vi "Manual Assembly DB.vi"() -> ()   [LabVIEW 2021]
uses:
  Classes/Routine/Routine Enum.ctl
  Classes/Assembly/Database Entry/Database Entry.lvclass
  Classes/Assembly/Assembly Run.lvclass
  Classes/Workspace/Fixture Enum.ctl
  Classes/Controller/Controller.lvclass
  Classes/Workspace/Fixture.lvclass
  Classes/Routine/Routine.lvclass
panel:
  in  "Type":bool
  out "String":string
  in  "Clear All":bool
  in  "Assemble":bool
  in  "Dispense offset":bool
  in  "Pick and Place":bool
  in  "Dispense glue":bool
  in  "Go":bool
  in  "Routine":T1=enum."Dispense on Plate"
  in  "Update":bool
  in  "Stage":i32(listbox)=-1
  in  "Stop":bool
  in  "Remove":bool
  in  "Add":bool
  # "Protomodule"
  # "Module"
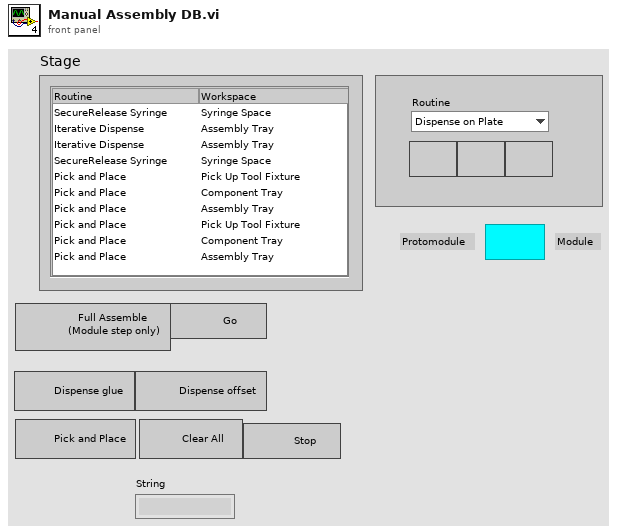
[diagram p1: front panel]
types:
  T1 = typedef "Routine.lvclass/Routine Enum.ctl" = enum16{"Primary Pick Up", "Pick Up All", "Put Down Secondary", "Put Down All", "Release Syringe", "Secondary Pick Up", "Secure Syringe", "Dispense on Plate", "Dispense on Kapton", "Dispense on Sensor"}
  T2 = typedef "Fixture.lvclass/Fixture Enum.ctl" = enum16{"Assembly Tray", "Syringe Space", "Component", "Pick Up Tool", "Current Position"}
  T3 = typedef "Controller.lvclass/Controllers.ctl" = cluster{"I-O.lvclass":refnum<class "I-O.lvclass">, "Gantry":refnum<k24>, "Dispenser":refnum<visa-resource-name>}
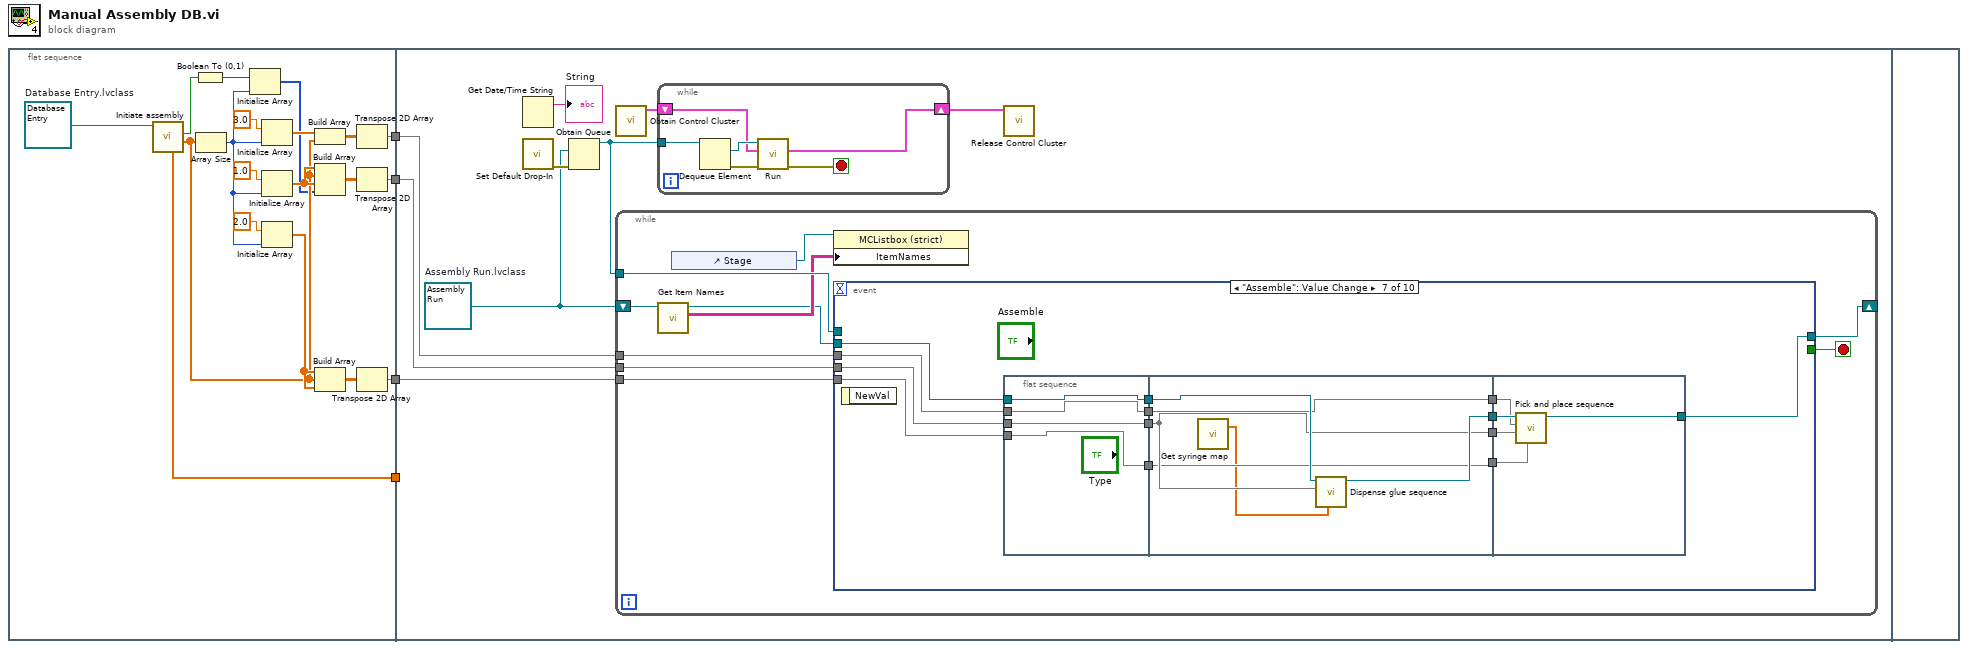
[diagram p0: block diagram]
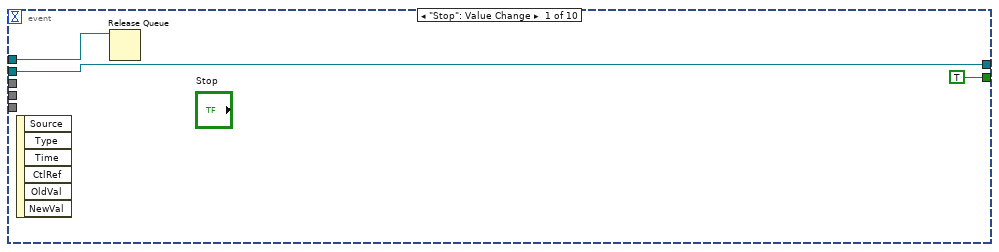
[diagram p2: hidden frame]
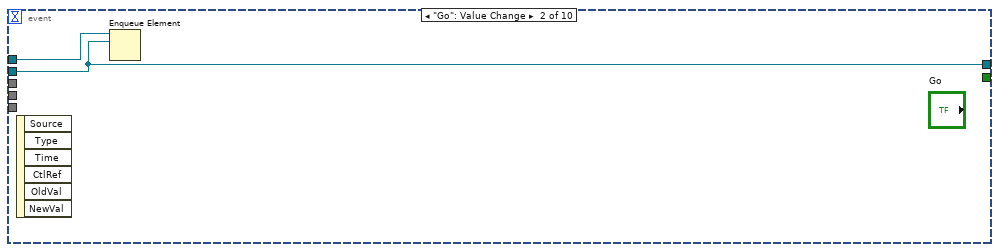
[diagram p3: hidden frame]
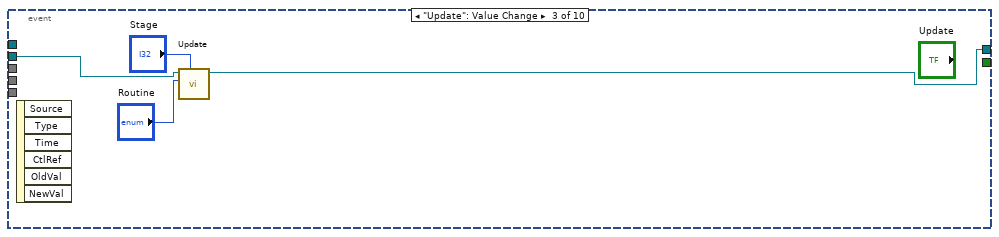
[diagram p4: hidden frame]
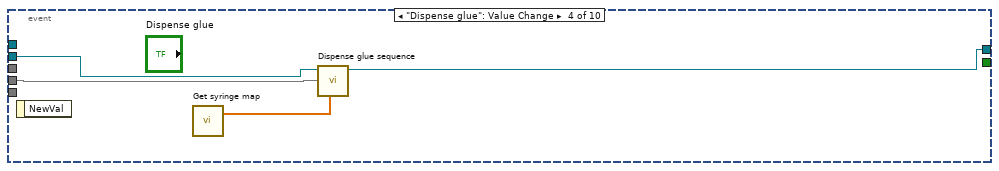
[diagram p5: hidden frame]
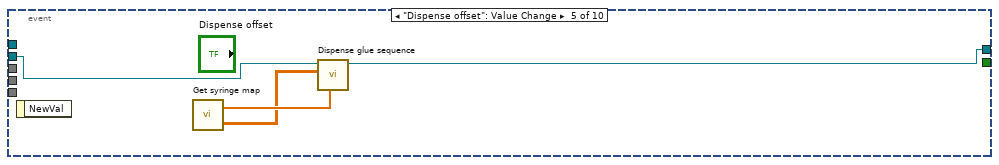
[diagram p6: hidden frame]
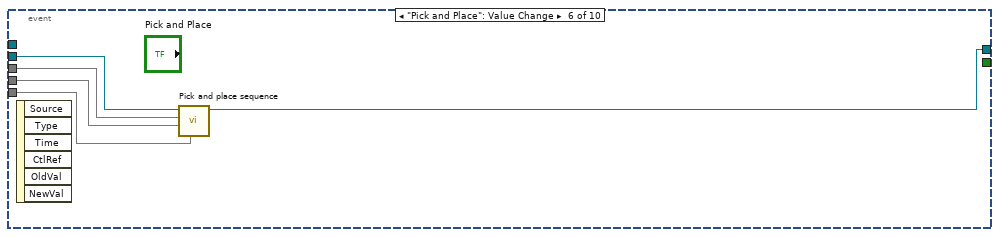
[diagram p7: hidden frame]
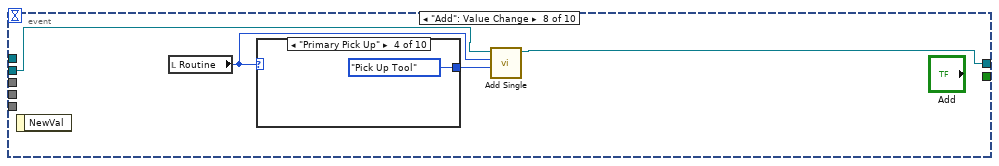
[diagram p8: hidden frame]
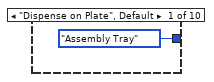
[diagram p9: hidden frame]
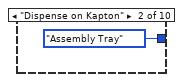
[diagram p10: hidden frame]
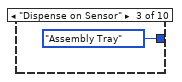
[diagram p11: hidden frame]
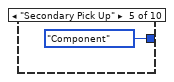
[diagram p12: hidden frame]
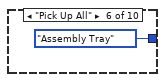
[diagram p13: hidden frame]
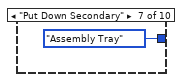
[diagram p14: hidden frame]
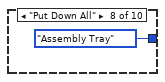
[diagram p15: hidden frame]
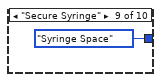
[diagram p16: hidden frame]
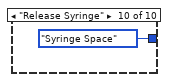
[diagram p17: hidden frame]
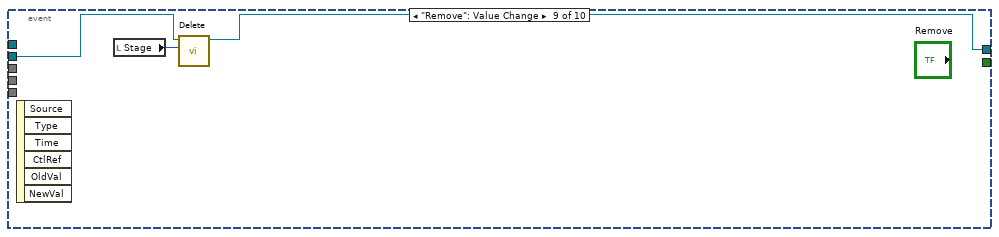
[diagram p18: hidden frame]
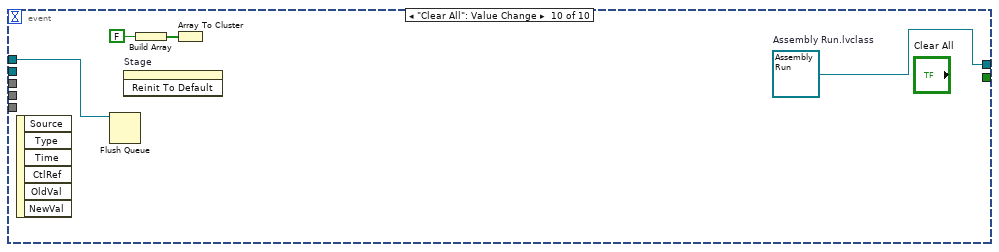
[diagram p19: hidden frame]
diagram:
  n1 = flat-sequence {
    tunnel: [w19] -> w4
    tunnel: [w15] -> w3
    tunnel: [w6] -> w2
    tunnel: [w5] -> w1
    tunnel: w4 -> [w26]
    tunnel: w3 -> [w25]
    tunnel: w2 -> [w24]
    tunnel: w1 -> [_]
    frame #0 {
      w23 = refnum<class "Database Entry.lvclass"> refnum  # Database Entry.lvclass
      n2 = call "Initiate assembly.vi"("Database Entry in"=w23) -> ("Selected postitions"=w11:dbl[], "Module?"=w8:bool, "Baselayer Thickness"=w5:dbl[])  [unwired: 6 in, 2 out]
      n3 = Boolean To (0,1)(Boolean=w8) -> (0, 1=w7:i16)
      n4 = Array Size(array=w11) -> (size(s)=w9:i32)
      n5 = Initialize Array(w7, w9) -> (w10:i16[])
      n6 = Initialize Array(3.0 ("element"), w9) -> (w21:dbl[])
      n7 = Initialize Array(1.0 ("element"), w9) -> (w12:dbl[])
      n8 = Initialize Array(2.0 ("element"), w9) -> (w16:dbl[])
      n9 = Build Array(w21, w11) -> (w20:dbl[][])
      n10 = Build Array(w12, w11, w12, w10) -> (w13:dbl[][])
      n11 = Build Array(w16, w11, w16) -> (w17:dbl[][])
      n12 = Transpose 2D Array(2D array=w20) -> (transposed array=w19:dbl[][])
      n13 = Transpose 2D Array(2D array=w13) -> (transposed array=w6:dbl[][])
      n14 = Transpose 2D Array(2D array=w17) -> (transposed array=w15:dbl[][])
    }
    frame #1 {
      w29 = refnum<class "Assembly Run.lvclass"> refnum  # Assembly Run.lvclass
      n15 = Get Date/Time String() -> (date string=→"String":string)  [unwired: 3 in, 1 out]
      n16 = call "Set Default Drop-In.vi"() -> ("error out"=w30:errorcluster)  [unwired: 11 in]
      n17 = Obtain Queue(element data type=w29, error in (no error)=w30) -> (queue out=w32:refnum<queue>)  [unwired: 3 in, 2 out]
      n18 = call "Obtain Control Cluster.vi"() -> ("Control Out"=w28:T3)  [unwired: 11 in]
      n19 = while {
        shift-right: [w36] -> _
        shift-left: w29 -> [w38]
        tunnel: w32 -> [w41]
        tunnel: w26 -> [w35]
        tunnel: w25 -> [w34]
        tunnel: w24 -> [w33]
        stop <- w42 stop-if-true
        n20 = call "Get Item Names.vi"("Assembly Run in"=w38) -> ("Item names"=w40:string[][], "Assembly Run out"=w37:refnum<class "Assembly Run.lvclass">)  [unwired: 8 in, 1 out]
        n21 = control-ref of="Stage"() -> (w39:refnum<vi>)
        n22 = property class="MCListbox (strict)"(reference=w39, "ItemNames"=w40) -> ()  [unwired: 1 in, 2 out]
        n23 = event shown="[6] \"Assemble\": Value Change" {
          selector: _ -> [_ _ _ _ _ _ _ _ _ _]
          dyn-events: _ -> [_ _ _ _ _ _ _ _ _ _]
          timeout: _ -> [_ _ _ _ _ _ _ _ _ _]
          tunnel: [TRUE _ _ _ _ _ _ _ _ _] -> w42
          tunnel: w37 -> [w44 w46 w51 w55 w59 w64 w77 w95 w109 _]
          tunnel: [w44 w46 w50 w54 w58 w63 w76 w94 w108 w113] -> w36
          tunnel: w41 -> [w43 w47 _ _ _ _ _ _ _ w112]
          tunnel: w35 -> [_ _ _ _ _ w62 w67 _ _ _]
          tunnel: w34 -> [_ _ _ _ _ w61 w66 _ _ _]
          tunnel: w33 -> [_ _ _ w52 _ w60 w65 _ _ _]
          event "Stop": Value Change {
            n24 = event-data() -> ()  [unwired: 1 in, 6 out]
            n25 = Release Queue(queue=w43) -> ()  [unwired: 2 in, 3 out]
          }
          event "Go": Value Change {
            n26 = event-data() -> ()  [unwired: 1 in, 6 out]
            n27 = Enqueue Element(queue=w47, element=w46) -> ()  [unwired: 2 in, 3 out]
          }
          event "Update": Value Change {
            n28 = event-data() -> ()  [unwired: 1 in, 6 out]
            n29 = call "Update.vi"("Row"="Stage", "Routine"="Routine", "Assembly Run in"=w51) -> ("Assembly Run out"=w50:refnum<class "Assembly Run.lvclass">)  [unwired: 7 in, 1 out]
          }
          event "Dispense glue": Value Change {
            n30 = event-data() -> ()  [unwired: 1 in, 1 out]
            n31 = call "Get syringe map.vi"() -> ("Syringe map"=w53:dbl[])  [unwired: 2 in, 1 out]
            n32 = call "Dispense glue sequence.vi"("Syringe map"=w53, "Assembly Tray map"=w52, "Assembly Run in"=w55) -> ("Assembly Run out"=w54:refnum<class "Assembly Run.lvclass">)  [unwired: 7 in, 1 out]
          }
          event "Dispense offset": Value Change {
            n33 = event-data() -> ()  [unwired: 1 in, 1 out]
            n34 = call "Get syringe map.vi"() -> ("Offset map (2D 1 row)"=w56:dbl[][], "Syringe map"=w57:dbl[])  [unwired: 2 in]
            n35 = call "Dispense glue sequence.vi"("Syringe map"=w57, "Assembly Tray map"=w56, "Assembly Run in"=w59) -> ("Assembly Run out"=w58:refnum<class "Assembly Run.lvclass">)  [unwired: 7 in, 1 out]
          }
          event "Pick and Place": Value Change {
            n36 = event-data() -> ()  [unwired: 1 in, 6 out]
            n37 = call "Pick and place sequence.vi"("Component Tray map"=w61, "Assembly Tray map"=w60, "PUT map"=w62, "Assembly Run in"=w64) -> ("Assembly Run out"=w63:refnum<class "Assembly Run.lvclass">)  [unwired: 6 in, 1 out]
          }
          event "Assemble": Value Change {
            n38 = event-data() -> ()  [unwired: 1 in, 1 out]
            n39 = flat-sequence {
              tunnel: [w81] -> w74
              tunnel: [w78] -> w73
              tunnel: [w79] -> w70
              tunnel: [w80] -> w68
              tunnel: w77 -> [w81]
              tunnel: w67 -> [w80]
              tunnel: w66 -> [w79]
              tunnel: w65 -> [w78]
              tunnel: [w86] -> w75
              tunnel: w74 -> [w87]
              tunnel: w73 -> [w85]
              tunnel: [w85] -> w72
              tunnel: [w84] -> w71
              tunnel: w70 -> [w84]
              tunnel: [w83] -> w69
              tunnel: w68 -> [w83]
              tunnel: [w91] -> w76
              tunnel: w75 -> [w92]
              tunnel: w72 -> [w90]
              tunnel: w71 -> [w89]
              tunnel: w69 -> [w88]
              frame #0 {
              }
              frame #1 {
                n40 = call "Get syringe map.vi"() -> ("Syringe map"=w82:dbl[])  [unwired: 2 in, 1 out]
                n41 = call "Dispense glue sequence.vi"("Syringe map"=w82, "Assembly Tray map"=w85, "Assembly Run in"=w87) -> ("Assembly Run out"=w86:refnum<class "Assembly Run.lvclass">)  [unwired: 7 in, 1 out]
              }
              frame #2 {
                n42 = call "Pick and place sequence.vi"("Component Tray map"=w89, "Assembly Tray map"=w90, "PUT map"=w88, "Assembly Run in"=w92) -> ("Assembly Run out"=w91:refnum<class "Assembly Run.lvclass">)  [unwired: 6 in, 1 out]
              }
            }
          }
          event "Add": Value Change {
            n43 = event-data() -> ()  [unwired: 1 in, 1 out]
            n44 = local read "Routine"() -> (w93:T1)
            n45 = case shown="\"Primary Pick Up\"" w93 {
              tunnel: [Fixture_Enum."Assembly Tray" ("Fixture") Fixture_Enum."Assembly Tray" ("Fixture") Fixture_Enum."Assembly Tray" ("Fixture") Fixture_Enum."Pick Up Tool" ("Fixture") Fixture_Enum."Component" ("Fixture") Fixture_Enum."Assembly Tray" ("Fixture") Fixture_Enum."Assembly Tray" ("Fixture") Fixture_Enum."Assembly Tray" ("Fixture") Fixture_Enum."Syringe Space" ("Fixture") Fixture_Enum."Syringe Space" ("Fixture")] -> w96
              frame "Dispense on Plate", Default {
              }
              frame "Dispense on Kapton" {
              }
              frame "Dispense on Sensor" {
              }
              frame "Primary Pick Up" {
              }
              frame "Secondary Pick Up" {
              }
              frame "Pick Up All" {
              }
              frame "Put Down Secondary" {
              }
              frame "Put Down All" {
              }
              frame "Secure Syringe" {
              }
              frame "Release Syringe" {
              }
            }
            n46 = call-dynamic "Add Single.vi"("Fixture"=w96, "Routine"=w93, "UI in"=w95) -> ("UI out"=w94:refnum<class "Assembly Run.lvclass">)  [unwired: 6 in, 1 out]
          }
          event "Remove": Value Change {
            n47 = event-data() -> ()  [unwired: 1 in, 6 out]
            n48 = local read "Stage"() -> (w107:i32)
            n49 = call "Delete.vi"("Index"=w107, "Assembly In"=w109) -> ("Assembly Out"=w108:refnum<class "Assembly Run.lvclass">)  [unwired: 8 in, 1 out]
          }
          event "Clear All": Value Change {
            w113 = refnum<class "Assembly Run.lvclass"> refnum  # Assembly Run.lvclass
            n50 = event-data() -> ()  [unwired: 1 in, 6 out]
            n51 = Flush Queue(queue=w112) -> ()  [unwired: 1 in, 3 out]
            n52 = invoke on="Stage" class="MCListbox (strict)" method="Reinit To Default"() -> ()  [unwired: 3 in, 3 out]
            n53 = Build Array(FALSE) -> (w111:bool[])
            n54 = Array To Cluster(array=w111) -> ()  [unwired: 1 out]
          }
        }
      }
      n55 = while {
        tunnel: w32 -> [w119]
        shift-right: [w114] -> w31
        shift-left: w28 -> [w115]
        stop <- w116 stop-if-true
        n56 = Dequeue Element(queue=w119) -> (element=w118:refnum<class "Assembly Run.lvclass">, error out=w117:errorcluster)  [unwired: 2 in, 2 out]
        n57 = call-dynamic "Run.vi"("error in (no error)"=w117, "Control In"=w115, "Assembly In"=w118) -> ("error out"=w116:errorcluster, "Control Out"=w114:T3)  [unwired: 6 in, 1 out]
      }
      n58 = call "Release Control Cluster.vi"("output cluster"=w31) -> ()  [unwired: 11 in]
    }
    frame #2 {
    }
  }
